vi "Statusword_ModeSpecific_ReferenceMove.vi"(11 "StatusWord In":u16 format="%08b") -> (0 "Set Point Reached?":bool, 3 "StatusWord Out":u16 format="%08b")   [LabVIEW 2017, in "WordManipulationLibrary.lvlib"]
uses:
  WordManipulationLibrary.lvlib
  Bit Manipulation.lvlib
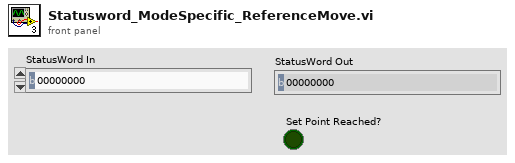
[diagram p1: front panel]
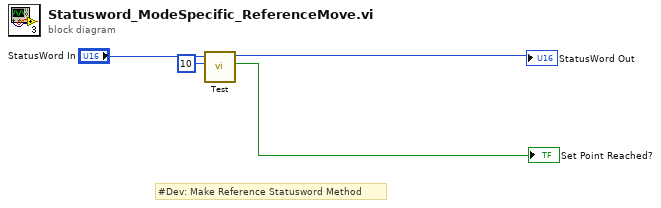
[diagram p0: block diagram]
diagram:
  # "#Dev: Make Reference Statusword Method"
  n1 = call "Test.vi"("Bit to test"=u8 10, "Data_In"="StatusWord In") -> ("bit value"=→"Set Point Reached?":bool, "Data_Out"=→"StatusWord Out":u16)  [unwired: 8 in]
